vi "Install LabVIEW Support.vi"() -> ()   [LabVIEW 2014, in "LMH-LINX.lvlib"]
uses:
  <vilib>/MakerHub/LINX/LMH-LINX.lvlib
  <vilib>/MakerHub/LINX/Private/Utilties/Target Management/Target Info.ctl
  <vilib>/MakerHub/LINX/Private/Utilties/Install LV Events.ctl
  <vilib>/MakerHub/LINX/Private/Utilties/Target Management/Install LV Data.ctl
  <vilib>/MakerHub/LINX/Private/Utilties/Target Management/Status FGV States.ctl
  <vilib>/Platform/browser.llb/Open URL in Default Browser (path).vi
  C:/Program Files (x86)/National Instruments/LabVIEW 2014/vi.lib/MakerHub/LINX/Resources/Renci.SshNet.dll
  vi.lib/MakerHub/LINX/Resources/Renci.SshNet.dll
  <vilib>/MakerHub/Toolbox/LMH-Toolbox.lvlib
panel:
  in  "Finish 2":bool
  in  "Finish":bool
  in  "Example":bool
  in  "Install":bool
  in  "Connect":bool
  in  "Password":string
  in  "Username":string="root"
  in  "Hostname or IP":string="192.168.7.2"
  out "Event Error":errorcluster
  out "Event Handler Iterations":i32
  out "Detailed Log":string
  out "Live Status":string
  out "Status Log":string
  out "Target Info":T1={"OS Version"="\n", "CPU"="", "Systemd Version"="", "Internet Access"=FALSE, "Device Type"=""}
  in  "View Log":bool
  out "EULA Link":string="here"
  out "Error Out":errorcluster
  # "The software installed by this wizard may be deployed on your hardware targets solely for your personal, \nnon-commercial use. Software is provided AS IS and with NO EXPRESS OR IMPLIED WARRANTIES.  \nThe full terms of the license can be found         ."
  # "Use this VI to install LabVIEW support to your BeagleBone Black or Raspberry Pi 2.\n\n1. Ensure the target is powered on, connected to this computer, and that the target has internet access.\n2. Enter the target's hostname or IP address.\n3. Enter the username and password for an account with sudo privileges on the target.\n          BBB defaults to 'root' and no password.\n          RPI2 running Raspbian defaults to 'pi' and 'raspberry'"
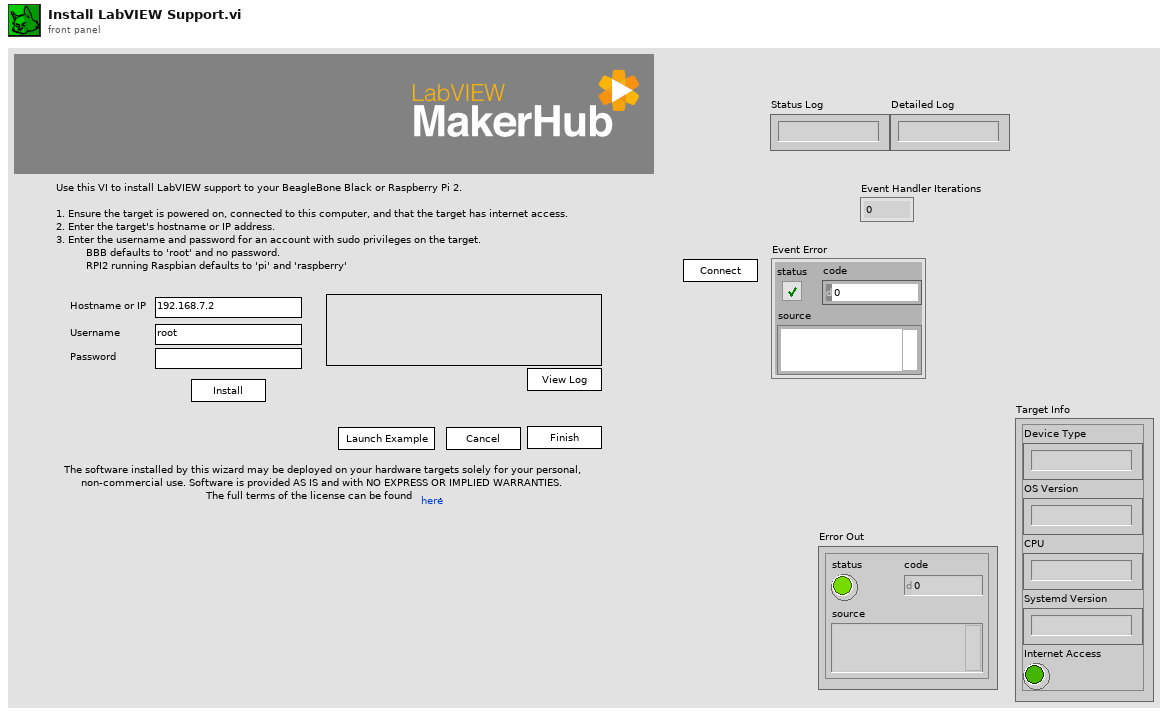
[diagram p1: front panel]
types:
  T1 = typedef "LMH-LINX.lvlib/Target Info.ctl" = cluster{"OS Version":string, "CPU":string, "Systemd Version":string, "Internet Access":bool, "Device Type":string}
  T2 = typedef "LMH-LINX.lvlib/Install LV Data.ctl" = cluster{"SSH Session":refnum<k24>, "Status Log":string, "Detailed Log":string, "Credentials":cluster{"Hostname or IP":string, "Username":string, "Password":string}, "Target Info":T1}
  T3 = typedef "LMH-LINX.lvlib/Install LV Events.ctl" = enum16{"Idle", "Connect", "Interrogate Device", "Add MakerHub Feed", "Update Package Index", "Install LV", "Start LV", "Launch Example", "View Log", "Exit"}
  T4 = typedef "LMH-LINX.lvlib/Status FGV States.ctl" = enum16{"Init", "Append", "Append History Only", "Set", "Get"}
  T5 = typedef "LMH-LINX.lvlib/Target Compatibility Warnings.ctl" = cluster{"Warning?":bool, "Details":string, "Help URL":string}
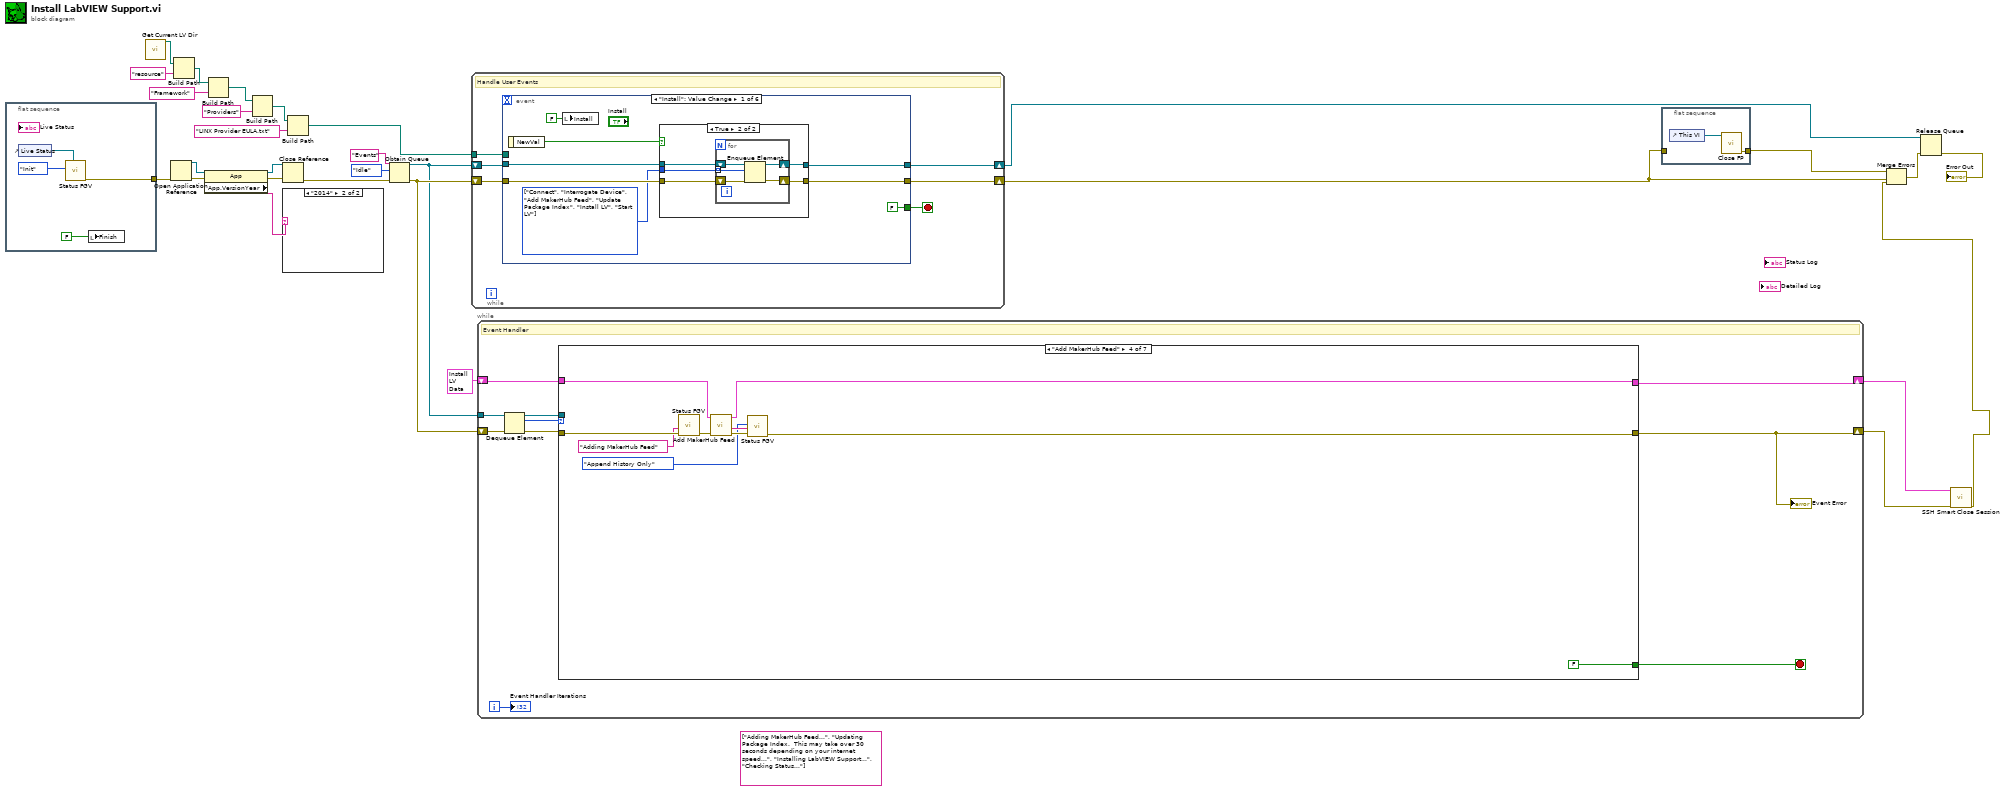
[diagram p0: block diagram]
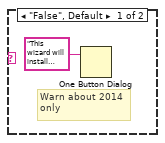
[diagram p2: hidden frame]
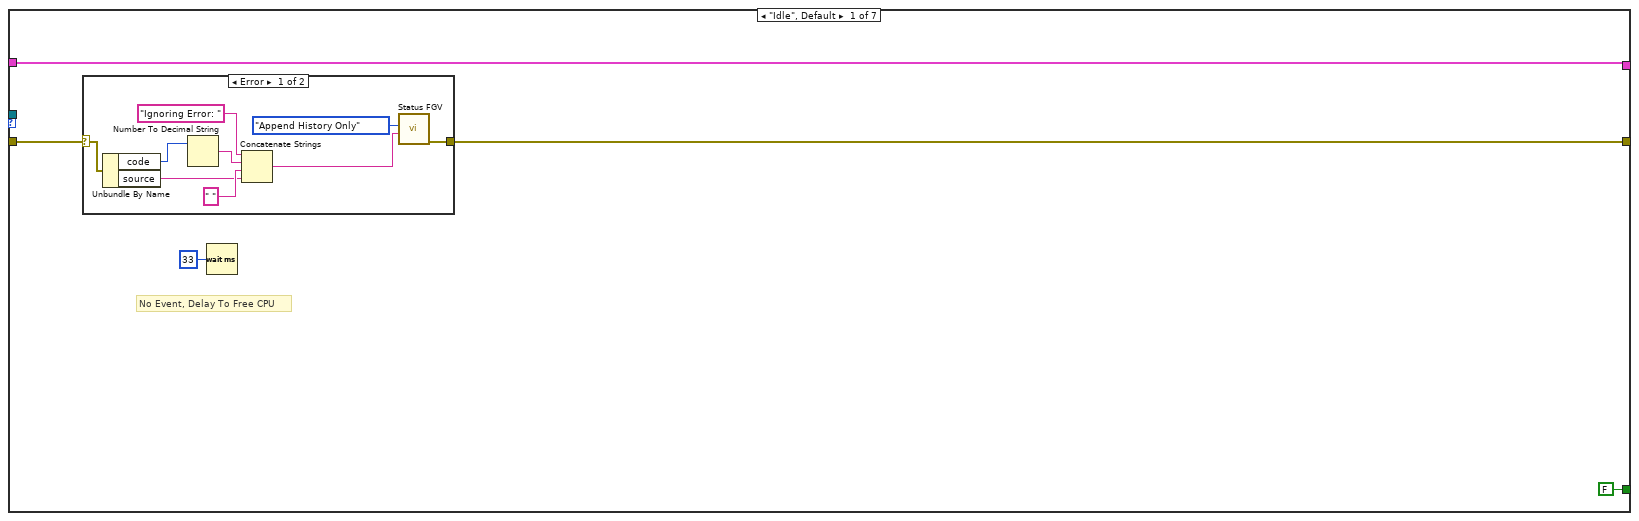
[diagram p3: hidden frame]
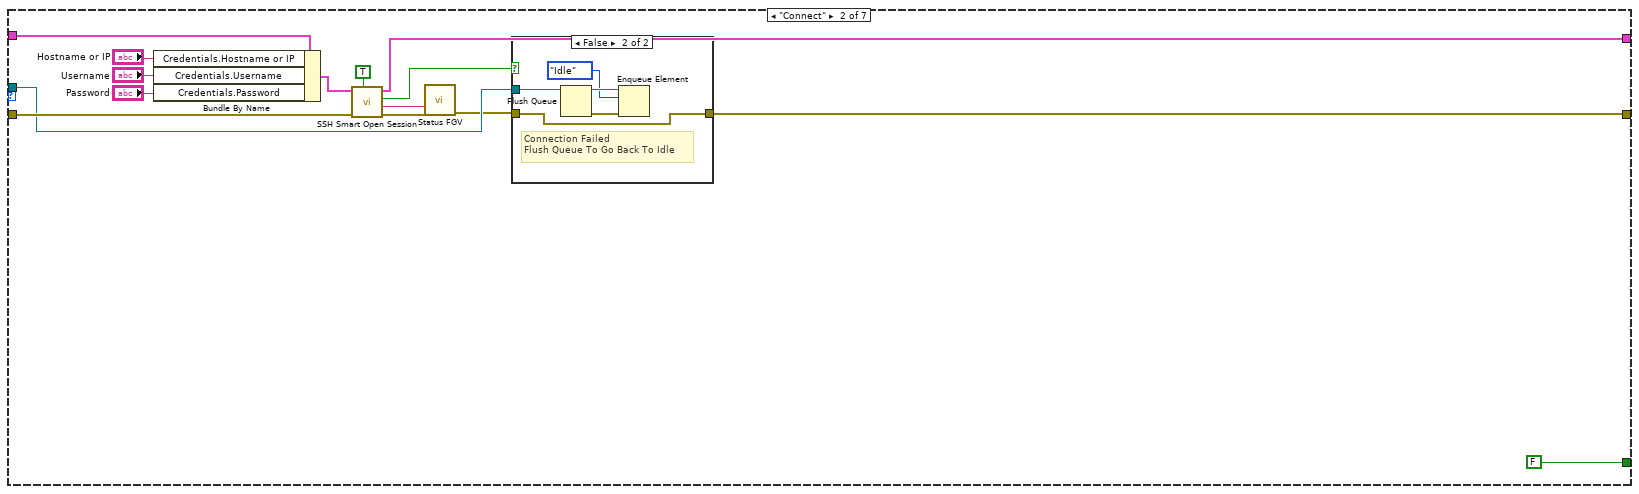
[diagram p5: hidden frame]
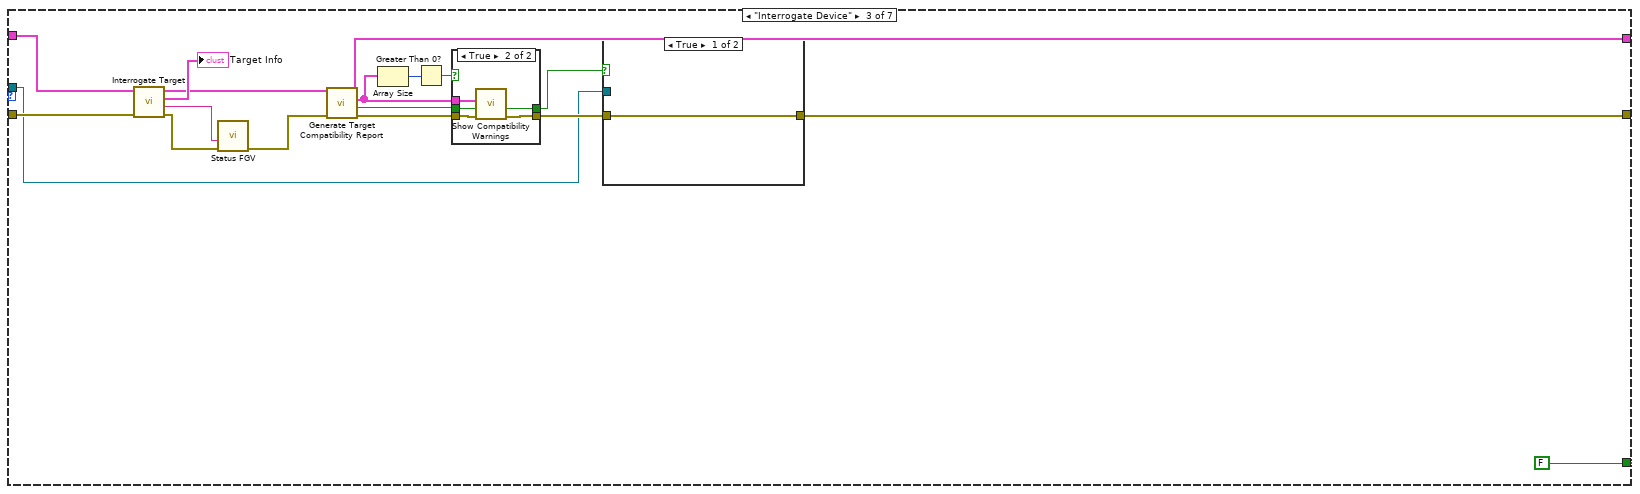
[diagram p7: hidden frame]
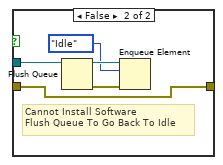
[diagram p8: hidden frame]
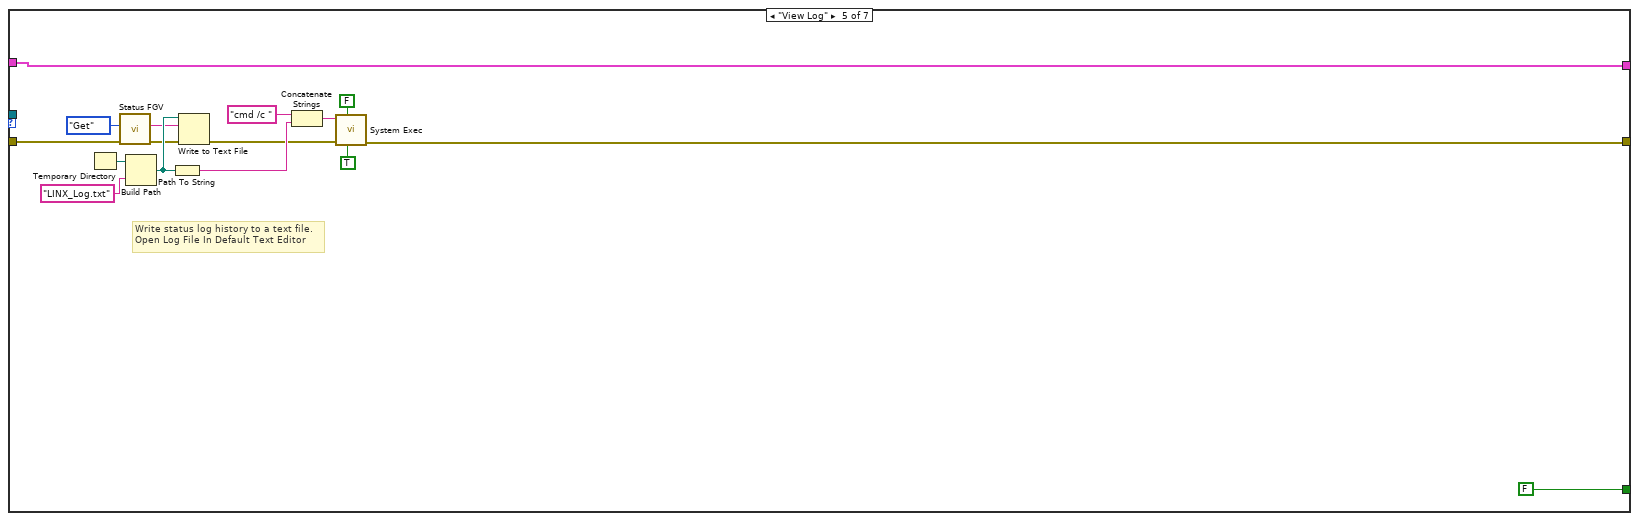
[diagram p10: hidden frame]
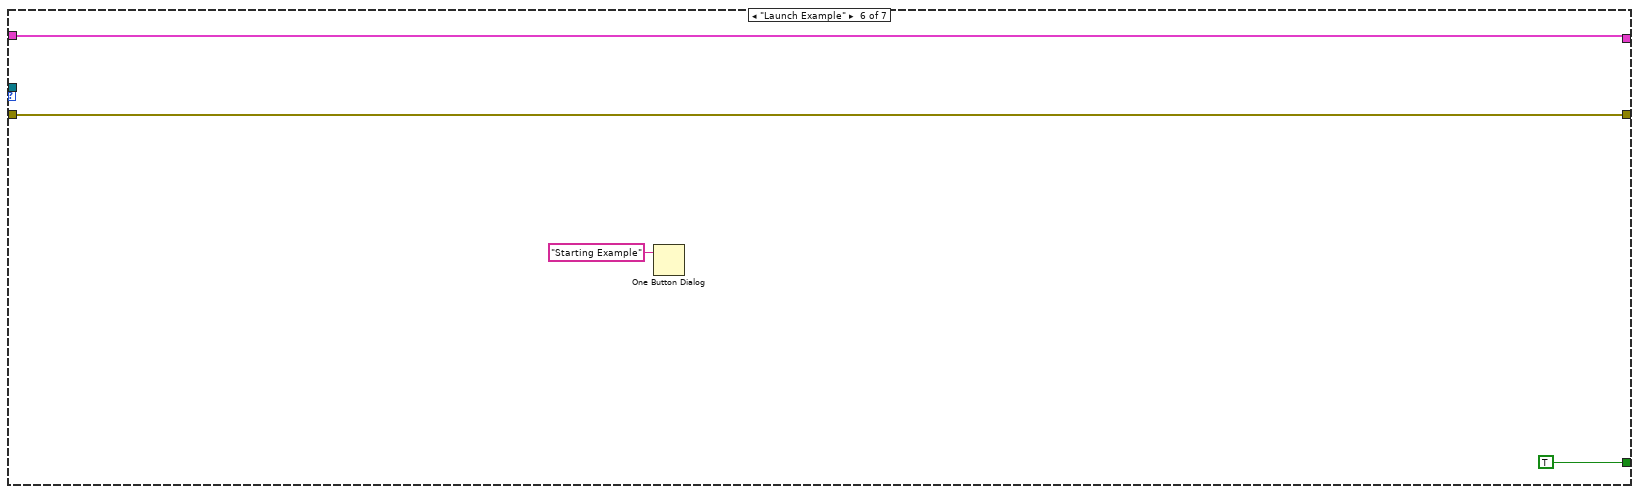
[diagram p11: hidden frame]
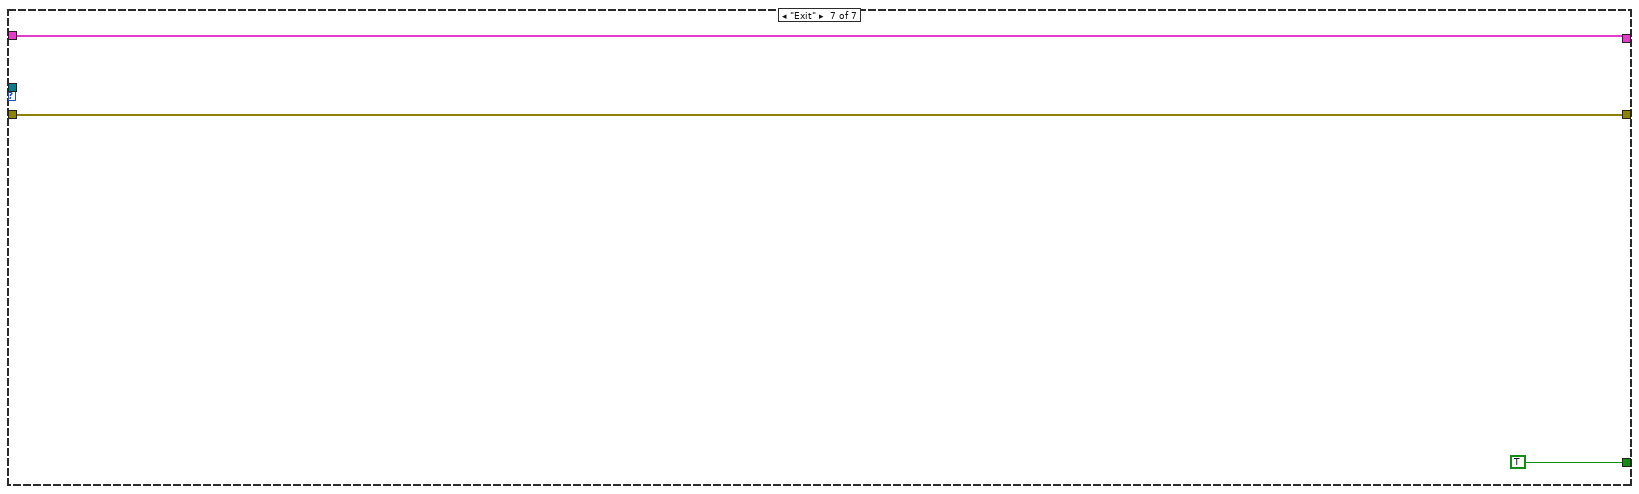
[diagram p12: hidden frame]
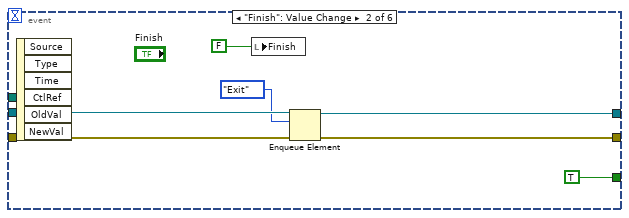
[diagram p14: hidden frame]
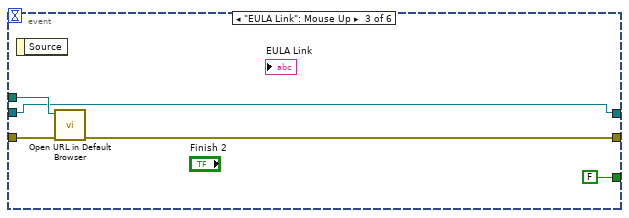
[diagram p15: hidden frame]
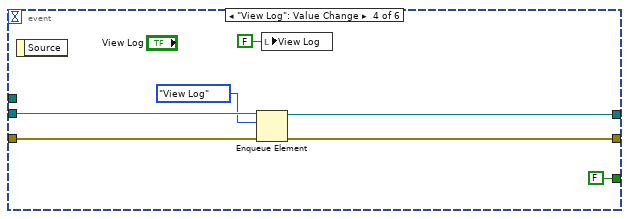
[diagram p16: hidden frame]
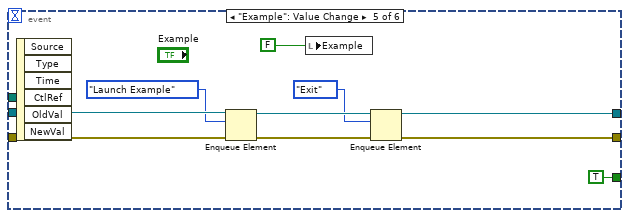
[diagram p17: hidden frame]
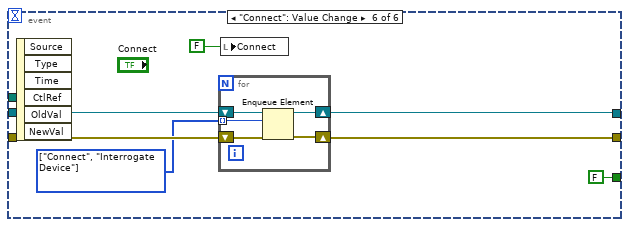
[diagram p18: hidden frame]
diagram:
  (unwired) string[] ["Adding MakerHub Feed...", "Updating Package Index.  This may take over 30 seconds depending on your internet speed...", "Installing LabVIEW Support...", "Checking Status..."]
  n1 = flat-sequence {
    tunnel: [w30] -> w1
    frame #0 {
      n2 = control-ref of="Live Status"() -> (w32:refnum<vi>)
      n3 = call <vilib>:"Status FGV.vi"("Live Status Ref"=w32, "Status FGV State"=Status_FGV_States."Init") -> ("Error Out"=w30:errorcluster)  [unwired: 7 in, 2 out]
      n4 = local write "Finish"(FALSE ("Stop Button")) -> ()
    }
  }
  n5 = call <vilib>:"Get Current LV Dir.vi"() -> ("This LV Directory"=w27:path)  [unwired: 10 in, 1 out]
  n6 = Open Application Reference(8:w1) -> (0:w17:errorcluster, 3:w14:refnum<vi>)  [unwired: 3 in]
  n7 = Build Path(base path=w27, name or relative path="resource") -> (appended path=w20:path)
  n8 = property class="App"(reference=w14, error in=w17) -> (reference out=w15:refnum<vi>, error out=w16:errorcluster, "App.VersionYear"=w18:string)
  n9 = Build Path(base path=w20, name or relative path="Framework") -> (appended path=w21:path)
  n10 = Build Path(base path=w21, name or relative path="Providers") -> (appended path=w22:path)
  n11 = Close Reference(reference=w15, error in (no error)=w16) -> (error out=w12:errorcluster)
  n12 = case shown="\"2014\"" w18 {
    frame "False", Default {
      # "Warn about 2014\nonly"
      n13 = One Button Dialog(message="This wizard will install LabVIEW 2014 support to the target device.  \nYou will only be able to connect to and use the device from LabVIEW 2014.") -> ()  [unwired: 1 in, 1 out]
    }
    frame "2014" {
    }
  }
  n14 = Build Path(base path=w22, name or relative path="LINX Provider EULA.txt") -> (appended path=w19:path)
  n15 = Obtain Queue(name (unnamed)="Events", element data type=Install_LV_Events."Idle" ("Install LV Support State"), error in (no error)=w12) -> (queue out=w10:refnum<queue>, error out=w11:errorcluster)  [unwired: 2 in, 1 out]
  n16 = while {
    shift-right: [w39] -> w28
    shift-left: w11 -> [w40]
    tunnel: w19 -> [w37]
    shift-right: [w36] -> w5
    shift-left: w10 -> [w35]
    stop <- w38 stop-if-true
    # "Handle User Events"
    n17 = event shown="[0] \"Install\": Value Change" {
      selector: _ -> [_ _ _ _ _ _]
      dyn-events: _ -> [_ _ _ _ _ _]
      timeout: _ -> [_ _ _ _ _ _]
      tunnel: [w45 w64 w72 w76 w80 w92] -> w39
      tunnel: w40 -> [w46 w65 w70 w77 w86 w91]
      tunnel: [FALSE TRUE FALSE FALSE TRUE FALSE] -> w38
      tunnel: w37 -> [_ _ w71 _ _ _]
      tunnel: [w43 w63 w68 w75 w81 w93] -> w36
      tunnel: w35 -> [w42 w62 w68 w74 w87 w94]
      event "Install": Value Change {
        w41 = T3[] [enum."Connect", enum."Interrogate Device", enum."Add MakerHub Feed", enum."Update Package Index", enum."Install LV", enum."Start LV"] items=["Idle", "Connect", "Interrogate Device", "Add MakerHub Feed", "Update Package Index", "Install LV", "Start LV", "Launch Example", "View Log", "Exit"]
        n18 = event-data() -> ("NewVal"=w44:bool)  [unwired: 1 in]
        n19 = local write "Install"(FALSE ("Install")) -> ()
        n20 = case shown="True" w44 {
          tunnel: w46 -> [w50 w55]
          tunnel: [w50 w54] -> w45
          tunnel: [w49 w53] -> w43
          tunnel: w42 -> [w49 w52]
          tunnel: w41 -> [_ w51]
          frame False {
            # "Ignore Change \nto False"
          }
          frame True {
            n21 = for {
              shift-right: [w59] -> w54
              shift-left: w55 -> [w60]
              shift-right: [w58] -> w53
              shift-left: w52 -> [w57]
              tunnel: w51 -> [w56] mode=indexing
              n22 = Enqueue Element(queue=w57, element=w56, error in (no error)=w60) -> (queue out=w58:refnum<queue>, error out=w59:errorcluster)  [unwired: 1 in, 1 out]
            }
          }
        }
      }
      event "Finish": Value Change {
        n23 = event-data() -> ()  [unwired: 1 in, 6 out]
        n24 = local write "Finish"(FALSE ("Stop Button")) -> ()
        n25 = Enqueue Element(queue=w62, element=Install_LV_Events."Exit", error in (no error)=w65) -> (queue out=w63:refnum<queue>, error out=w64:errorcluster)  [unwired: 1 in, 1 out]
      }
      event "EULA Link": Mouse Up {
        n26 = event-data() -> ()  [unwired: 1 in, 1 out]
        n27 = call-poly <vilib>:"Open URL in Default Browser.vi"("error in (no error)"=w70, "path"=w71) -> ("error out"=w72:errorcluster)  [unwired: 4 in, 1 out]
      }
      event "View Log": Value Change {
        n28 = event-data() -> ()  [unwired: 1 in, 1 out]
        n29 = Enqueue Element(queue=w74, element=Install_LV_Events."View Log", error in (no error)=w77) -> (queue out=w75:refnum<queue>, error out=w76:errorcluster)  [unwired: 1 in, 1 out]
        n30 = local write "View Log"(FALSE ("View Log")) -> ()
      }
      event "Example": Value Change {
        n31 = event-data() -> ()  [unwired: 1 in, 6 out]
        n32 = Enqueue Element(queue=w87, element=Install_LV_Events."Launch Example" ("Install LV Support State"), error in (no error)=w86) -> (queue out=w83:refnum<queue>, error out=w84:errorcluster)  [unwired: 1 in, 1 out]
        n33 = local write "Example"(FALSE ("Launch Example")) -> ()
        n34 = Enqueue Element(queue=w83, element=Install_LV_Events."Exit" ("Install LV Support State"), error in (no error)=w84) -> (queue out=w81:refnum<queue>, error out=w80:errorcluster)  [unwired: 1 in, 1 out]
      }
      event "Connect": Value Change {
        w90 = T3[] [enum."Connect", enum."Interrogate Device"] items=["Idle", "Connect", "Interrogate Device", "Add MakerHub Feed", "Update Package Index", "Install LV", "Start LV", "Launch Example", "View Log", "Exit"]
        n35 = event-data() -> ()  [unwired: 1 in, 6 out]
        n36 = for {
          shift-right: [w100] -> w92
          shift-left: w91 -> [w101]
          shift-right: [w99] -> w93
          shift-left: w94 -> [w98]
          tunnel: w90 -> [w97] mode=indexing
          n37 = Enqueue Element(queue=w98, element=w97, error in (no error)=w101) -> (queue out=w99:refnum<queue>, error out=w100:errorcluster)  [unwired: 1 in, 1 out]
        }
        n38 = local write "Connect"(FALSE ("Interrogate")) -> ()
      }
    }
  }
  n39 = while {
    shift-right: [w110] -> w2
    shift-left: w11 -> [w108]
    tunnel: w10 -> [w109]
    shift-right: [w105] -> w4
    shift-left: T2 {"SSH Session"=refnum, "Status Log"="", "Detailed Log"="", "Credentials"={"Hostname or IP"="192.168.7.2", "Username"="root", "Password"=""}, "Target Info"={"OS Version"="", "CPU"="", "Systemd Version"="", "Internet Access"=FALSE, "Device Type"=""}} ("Install LV Data") -> [w103]
    i -> [w104]
    stop <- w111 stop-if-true
    # "Event Handler"
    n40 = Dequeue Element(queue=w109, error in (no error)=w108) -> (queue out=w102:refnum<queue>, element=w106:T3, error out=w107:errorcluster)  [unwired: 1 in, 1 out]
    n41 = case shown="\"Add MakerHub Feed\"" w106 {
      tunnel: [w112 w133 w151 w179 w198 w207 w210] -> w110
      tunnel: w107 -> [w113 w141 w164 w187 w192 w207 w210]
      tunnel: [FALSE FALSE FALSE FALSE FALSE TRUE TRUE] -> w111
      tunnel: [w115 w140 w152 w180 w195 w205 w209] -> w105
      tunnel: w103 -> [w115 w136 w162 w181 w195 w205 w209]
      tunnel: w102 -> [_ w134 w149 _ _ _ _]
      frame "Idle", Default {
        # "No Event, Delay To Free CPU"
        n42 = case shown="Error" w113 {
          selector: w113 -> [w124 w126]
          tunnel: [w125 w126] -> w112
          frame Error {
            n43 = Unbundle By Name(w124) -> ("code"=w122:i32, "source"=w119:string)
            n44 = Number To Decimal String(number=w122) -> (decimal integer string=w121:string)  [unwired: 1 in]
            n45 = Concatenate Strings("Ignoring Error: " ("Status"), w121, " " ("string"), w119) -> (w118:string)
            n46 = call <vilib>:"Status FGV.vi"("Status"=w118, "Status FGV State"=Status_FGV_States."Append History Only") -> ("Error Out"=w125:errorcluster)  [unwired: 7 in, 2 out]
          }
          frame No Error {
          }
        }
        n47 = Wait (ms)(milliseconds to wait=u32 33) -> ()  [unwired: 1 out]
      }
      frame "Connect" {
        n48 = Bundle By Name(cluster=w136, "Credentials.Hostname or IP"="Hostname or IP", "Credentials.Username"="Username", "Credentials.Password"="Password") -> (w137:T2)
        n49 = call <vilib>:"SSH Smart Open Session.vi"("Force Reconnect?"=TRUE, "Error In"=w141, "Install LV Data in"=w137) -> ("Error Out"=w132:errorcluster, "Status"=w130:string, "Connected?"=w135:bool, "Install LV Data out"=w140:T2)  [unwired: 5 in]
        n50 = call <vilib>:"Status FGV.vi"("Error In"=w132, "Status"=w130) -> ("Error Out"=w131:errorcluster)  [unwired: 7 in, 2 out]
        n51 = case shown="False" w135 {
          tunnel: w134 -> [_ w147]
          tunnel: w131 -> [w142 w143]
          tunnel: [w142 w143] -> w133
          frame True {
          }
          frame False {
            # "Connection Failed\nFlush Queue To Go Back To Idle"
            n52 = Flush Queue(queue=w147) -> (queue out=w145:refnum<queue>, error out=w146:errorcluster)  [unwired: 1 in, 1 out]
            n53 = Enqueue Element(queue=w145, element=Install_LV_Events."Idle", error in (no error)=w146) -> ()  [unwired: 1 in, 3 out]
          }
        }
      }
      frame "Interrogate Device" {
        n54 = call <vilib>:"Interrogate Target.vi"("Error In"=w164, "Install LV Data"=w162) -> ("Error Out"=w161:errorcluster, "Status"=w160:string, "Target Info"=→"Target Info":T1, "Install LV Data"=w158:T2)  [unwired: 6 in]
        n55 = call <vilib>:"Status FGV.vi"("Error In"=w161, "Status"=w160) -> ("Error Out"=w159:errorcluster)  [unwired: 7 in, 2 out]
        n56 = call <vilib>:"Generate Target Compatibility Report.vi"("Error In"=w159, "Install LV Data"=w158) -> ("Error Out"=w157:errorcluster, "Can Continue?"=w156:bool, "Warnings"=w155:T5[], "Install LV Data"=w152:T2)  [unwired: 6 in]
        n57 = Array Size(array=w155) -> (size(s)=w154:i32)
        n58 = Greater Than 0?(x=w154) -> (x > 0?=w153:bool)
        n59 = case shown="True" w153 {
          tunnel: w157 -> [w173 w178]
          tunnel: [w173 w177] -> w150
          tunnel: w156 -> [w172 w176]
          tunnel: w155 -> [_ w175]
          tunnel: [w172 w174] -> w148
          frame False {
          }
          frame True {
            n60 = call <vilib>:"Show Compatibility Warnings.vi"("Error In"=w178, "Can Continue?"=w176, "Warnings"=w175) -> ("Error Out"=w177:errorcluster, "Continue?"=w174:bool)  [unwired: 7 in]
          }
        }
        n61 = case shown="True" w148 {
          tunnel: w149 -> [_ w171]
          tunnel: w150 -> [w166 w167]
          tunnel: [w166 w167] -> w151
          frame True {
          }
          frame False {
            # "Cannot Install Software\nFlush Queue To Go Back To Idle"
            n62 = Flush Queue(queue=w171) -> (queue out=w169:refnum<queue>, error out=w170:errorcluster)  [unwired: 1 in, 1 out]
            n63 = Enqueue Element(queue=w169, element=Install_LV_Events."Idle", error in (no error)=w170) -> ()  [unwired: 1 in, 3 out]
          }
        }
      }
      frame "Add MakerHub Feed" {
        n64 = call <vilib>:"Status FGV.vi"("Error In"=w187, "Status"="Adding MakerHub Feed") -> ("Error Out"=w186:errorcluster)  [unwired: 7 in, 2 out]
        n65 = call <vilib>:"Add MakerHub Feed.vi"("Error In"=w186, "Install LV Data"=w181) -> ("Error Out"=w184:errorcluster, "Log"=w183:string, "Install LV Data"=w180:T2)  [unwired: 7 in]
        n66 = call <vilib>:"Status FGV.vi"("Error In"=w184, "Status"=w183, "Status FGV State"=Status_FGV_States."Append History Only") -> ("Error Out"=w179:errorcluster)  [unwired: 6 in, 2 out]
      }
      frame "View Log" {
        # "Write status log history to a text file.\nOpen Log File In Default Text Editor"
        n67 = Temporary Directory() -> (w204:path)
        n68 = call <vilib>:"Status FGV.vi"("Error In"=w192, "Status FGV State"=Status_FGV_States."Get") -> ("Error Out"=w191:errorcluster, "History"=w189:string)  [unwired: 7 in, 1 out]
        n69 = Build Path(base path=w204, name or relative path="LINX_Log.txt") -> (appended path=w194:path)
        n70 = Path To String(path=w194) -> (string=w199:string)
        n71 = Write to Text File(file (use dialog)=w194, text=w189, error in=w191) -> (error out=w193:errorcluster)  [unwired: 1 in, 2 out]
        n72 = Concatenate Strings("cmd /c " ("command line"), w199) -> (w202:string)
        n73 = call <vilib>:"System Exec.vi"("run minimized? (F)"=TRUE, "wait until completion? (T)"=FALSE, "error in (no error)"=w193, "command line"=w202) -> ("error out"=w198:errorcluster)  [unwired: 4 in, 3 out]
      }
      frame "Launch Example" {
        n74 = One Button Dialog(message="Starting Example") -> ()  [unwired: 1 in, 1 out]
      }
      frame "Exit" {
      }
    }
    "Event Error" <- w110
    "Event Handler Iterations" <- w104
  }
  n75 = flat-sequence {
    tunnel: [w212] -> w29
    tunnel: w28 -> [_]
    frame #0 {
      n76 = control-ref of="This VI"() -> (w213:refnum<vi>)
      n77 = call <vilib>:"Close FP.vi"("VI Ref"=w213) -> ("Error Out"=w212:errorcluster)  [unwired: 10 in]
    }
  }
  n78 = call <vilib>:"SSH Smart Close Session.vi"("Error In"=w2, "Install LV Data"=w4) -> ("Error Out"=w3:errorcluster)  [unwired: 8 in, 1 out]
  n79 = Merge Errors(w29, w28, w3) -> (w7:errorcluster)
  n80 = Release Queue(queue=w5, error in (no error)=w7) -> (error out=→"Error Out":errorcluster)  [unwired: 1 in, 2 out]
